vi "SD-FindElement.vi"(8 "offset (0)":i32, 11 "XML String In":string) -> (0 "offset past match":i32, 1 "after  tag":string, 2 "tag":string, 3 "before tag":string, 5 "element name":string)   [LabVIEW 2020]
doc: "This VI finds the first XML start tag in the string and returns:\n\nbefore tag - portion of string prior to the tag\ntag - the contents of the tag including angle brackets (<,>)\nafter tag - portion of string found after the end of the tag\noffset past match - index in string of the first character of after substring\nelement name - the name (including namespace if applicable) of the element"
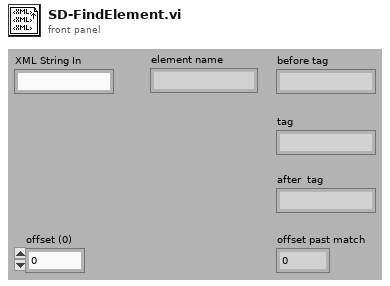
[diagram p1: front panel]
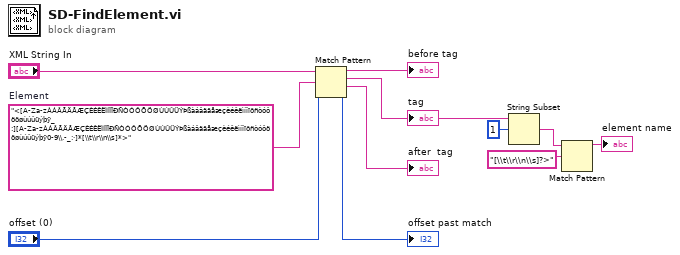
[diagram p0: block diagram]
diagram:
  w10 = "<[A-Za-zÀÁÂÃÄÅÆÇÈÉÊËÌÍÎÏÐÑÒÓÔÕÖØÙÚÛÜÝÞßàáâãäåæçèéêëìíîïðñòóôõöøùúûüýþÿ_:][A-Za-zÀÁÂÃÄÅÆÇÈÉÊËÌÍÎÏÐÑÒÓÔÕÖØÙÚÛÜÝÞßàáâãäåæçèéêëìíîïðñòóôõöøùúûüýþÿ0-9\\.-_:·]*[\\t\\r\\n\\s]*>"  # Element
  n1 = Match Pattern(string="XML String In", regular expression=w10, offset (0)="offset (0)") -> (before substring=→"before tag":string, match substring=w1:string, after substring=→"after  tag":string, offset past match=→"offset past match":i32)
  "tag" <- w1
  n2 = String Subset(string=w1, offset (0)=1) -> (substring=w2:string)  [unwired: 1 in]
  n3 = Match Pattern(string=w2, regular expression="[\\t\\r\\n\\s]?>") -> (before substring=→"element name":string)  [unwired: 1 in, 3 out]
